vi "Destroy.vi"(8 "error in (no error)":errorcluster, 11 "CameraManager":refnum<data-value>) -> (0 "error out":errorcluster)   [LabVIEW 2020, in "g_ar_toolkit.capture.lvlib" / "CameraManager.lvclass"]
uses:
  CameraManager.lvclass
  CameraManager.lvclass/CameraManager.ctl
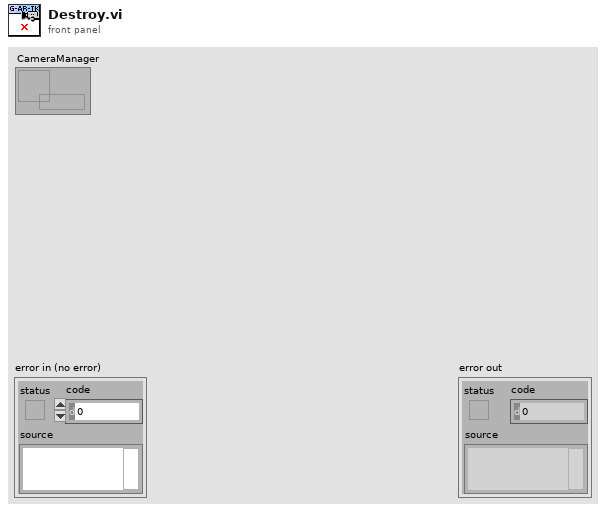
[diagram p1: front panel]
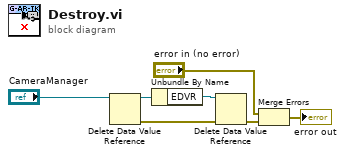
[diagram p0: block diagram]
diagram:
  n1 = Delete Data Value Reference(data value reference="CameraManager") -> (data value=w6:refnum<class "CameraManager.lvclass">, error out=w4:errorcluster)  [unwired: 1 in]
  n2 = Unbundle By Name(w6) -> ("EDVR"=w3:refnum<data-value>)
  n3 = Delete Data Value Reference(data value reference=w3, error in=w4) -> (error out=w2:errorcluster)  [unwired: 1 out]
  n4 = Merge Errors("error in (no error)", w2) -> (→"error out":errorcluster)
